vi "TopasError.vi"(8 "error in":errorcluster, 11 "Error Code":u64) -> (0 "error out":errorcluster)   [LabVIEW 2019, in "Topas.lvlib"]
uses:
  Topas.lvlib
  ErrorType.ctl
panel:
  in  "ErrorType":T1
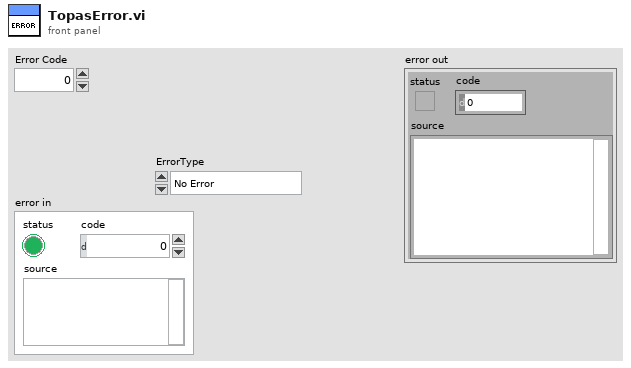
[diagram p1: front panel]
types:
  T1 = typedef "ErrorType.ctl" = enum16{"No Error", "Unknown Error", "No Topas USB device", "Invalid Device Instance", "Invalid device index", "Buffer too small", "Failed to get Topas USB serial number", "Device already opened", "Device failed to open", "USB communication channel failed to open", "USB read error", "Motor configuration failed to load", "Config file does not match config on board", "Transmitting parameters failed", "Device with this serial number not found", "Invalid interface card type", "Device is not opened", "USB command failed to receive response", "Wavelength can not be set ", "Invalid motor index", "Function is not supported by LPT card", "Invalid wavelength code", "Invalid unit code", "Tuning curve file failed to load", "Tuning curve file read error", "Wrong tuning curve file version", "Wrong tuning curve type", "Invalid number of motors", "Invalid number of interactions", "OPA type mismatch", "Invalid wavelength", "Invalid grating motor index in OPA tuning file", "Tuning curve type mismatch", "Configuration file not found"}
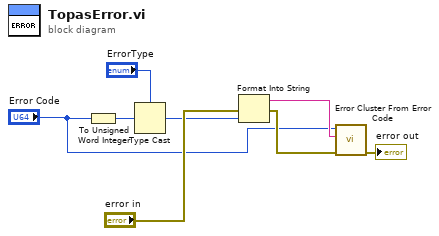
[diagram p0: block diagram]
diagram:
  n1 = To Unsigned Word Integer(number="Error Code") -> (unsigned 16bit integer=w1:u16)
  n2 = Type Cast(type="ErrorType", x=w1) -> (*(type *) &x=w3:T1)
  n3 = Format Into String(error in="error in", w3) -> (resulting string=w8:string, error out=w7:errorcluster)  [unwired: 2 in]
  n4 = call <vilib>:"Error Cluster From Error Code.vi"("error in (no error)"=w7, "error message (\"\")"=w8, "error code (0)"="Error Code") -> ("error out"=→"error out":errorcluster)  [unwired: 6 in]
